vi "Read settings.vi"(8 "error in (no error)":errorcluster, 11 "Counter in":refnum<class "Counter.lvclass">) -> (0 "error out":errorcluster, 2 "Counter Settings":T1 {"Array of Counter Settings"."clock rate (Hz)" format="%0.2f"}, 3 "Counter out":refnum<class "Counter.lvclass">)   [LabVIEW 2014, in "Counter.lvclass"]
uses:
  Counter.lvclass
  Counter_Settings_Control.ctl
  Counter.lvclass/Counter.ctl
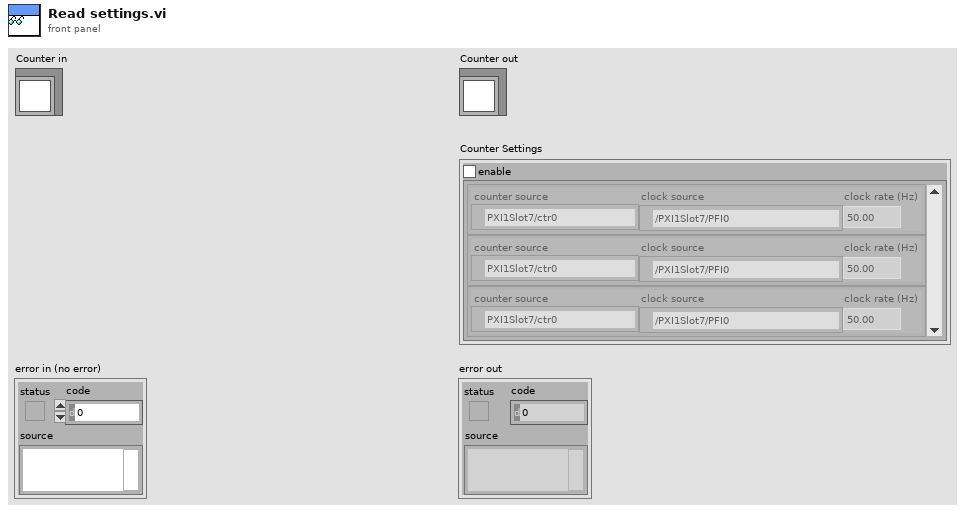
[diagram p1: front panel]
types:
  T1 = typedef "Counter.lvclass/Counter_Settings_Control.ctl" = cluster{"enable":bool, "Array of Counter Settings":cluster{"counter source":tag, "clock source":tag, "clock rate (Hz)":dbl}[]}
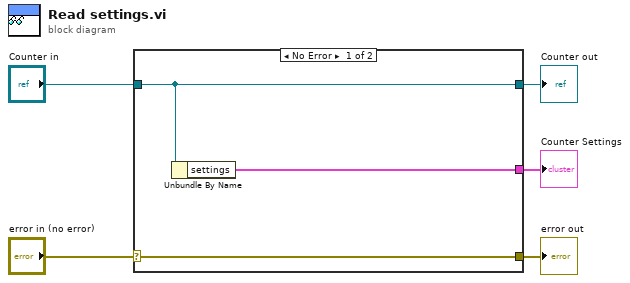
[diagram p0: block diagram]
diagram:
  n1 = case shown="No Error" "error in (no error)" {
    selector: "error in (no error)" -> [w8 w9]
    tunnel: [w8 w9] -> w4
    tunnel: [w7 w10] -> w2
    tunnel: "Counter in" -> [w7 w10]
    tunnel: [w6 _] -> w1
    frame No Error {
      n2 = Unbundle By Name(w7) -> ("settings"=w6:T1)
    }
    frame Error {
    }
  }
  "error out" <- w4
  "Counter out" <- w2
  "Counter Settings" <- w1
